vi "MGI Add Error[].vi"(8 "error in (no error)":errorcluster, 10 "Error[]":errorcluster[](array[cluster]), 11 "MGI Error Handler in":refnum<class "MGI Error Reporter Dialog.lvclass">) -> (0 "error out":errorcluster, 3 "MGI Error Handler out":refnum<class "MGI Error Reporter Dialog.lvclass">)   [LabVIEW 2016, in "MGI Error Reporter Dialog.lvclass"]
doc: "Add the errors in the specified array to the History Listbox. A child class may override this VI, which stores errors by process date and time (from most recent to oldest).\n\nAuthored by Shawn Walpole\nsupport@mooregoodideas.com\nwww.mooregoodideas.com\n\nCopyright (c) 2010, Moore Good Ideas, Inc.\n\nAll rights reserved.\n\nRedistribution and use in source and binary forms, with or without modification, are permitted provided that the following conditions are met:\n\n * Redistributions of source code must retain the above copyright notice, this list of conditions and the following disclaimer.\n * Redistributions in binary form must reproduce the above copyright notice, this list of conditions and the following disclaimer in the documentation and/or other materials provided with the distribution.\n * Neither the name of Moore Good Ideas, Inc. nor the names of its contributors may be used to endorse or promote products derived from this software without specific prior written permission.\n\nTHIS SOFTWARE IS PROVIDED BY THE COPYRIGHT HOLDERS AND CONTRIBUTORS \"AS IS\" AND ANY EXPRESS OR IMPLIED WARRANTIES, INCLUDING, BUT NOT LIMITED TO, THE IMPLIED WARRANTIES OF MERCHANTABILITY AND FITNESS FOR A PARTICULAR PURPOSE ARE DISCLAIMED. IN NO EVENT SHALL THE COPYRIGHT OWNER OR CONTRIBUTORS BE LIABLE FOR ANY DIRECT, INDIRECT, INCIDENTAL, SPECIAL, EXEMPLARY, OR CONSEQUENTIAL DAMAGES (INCLUDING, BUT NOT LIMITED TO, PROCUREMENT OF SUBSTITUTE GOODS OR SERVICES; LOSS OF USE, DATA, OR PROFITS; OR BUSINESS INTERRUPTION) HOWEVER CAUSED AND ON ANY THEORY OF LIABILITY, WHETHER IN CONTRACT, STRICT LIABILITY, OR TORT (INCLUDING NEGLIGENCE OR OTHERWISE) ARISING IN ANY WAY OUT OF THE USE OF THIS SOFTWARE, EVEN IF ADVISED OF THE POSSIBILITY OF SUCH DAMAGE."
uses:
  <userlib>/_MGI/Error Reporter/MGI Error Reporter Dialog/MGI Error Reporter Dialog.lvclass
  <userlib>/_MGI/Application Control/MGI Set Scrollbar/MGI Set Multicolumn Listbox Scrollbar.vi
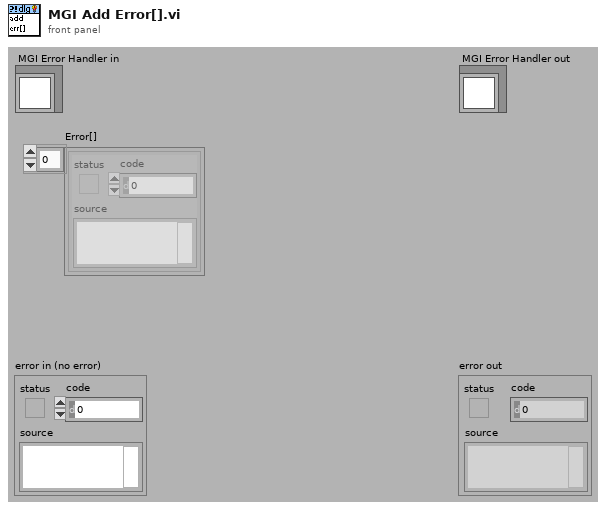
[diagram p1: front panel]
types:
  T1 = typedef "MGI Error Reporter Dialog.lvclass/MGI Dialog UI Refs Cluster.ctl" = cluster{"LB Ref":refnum<vi>, "Details Ref":refnum<vi>, "Caller Ring Ref":refnum<vi>, "Message Ref":refnum<vi>, "Clear Btn Ref":refnum<vi>}
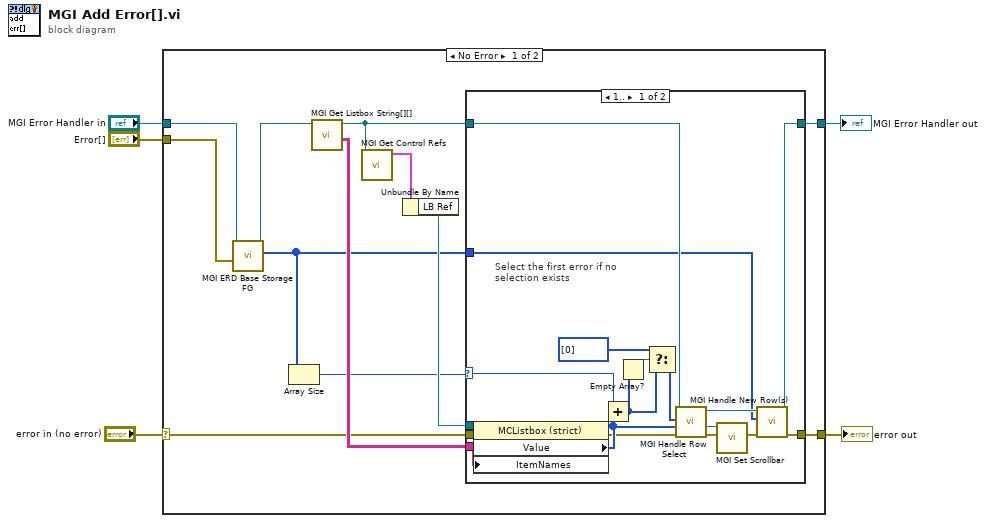
[diagram p0: block diagram]
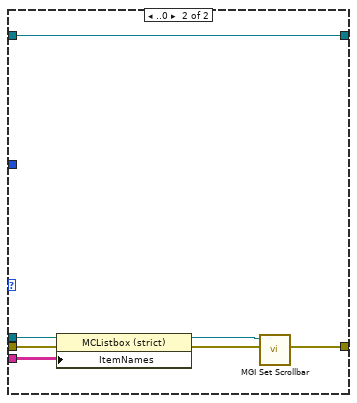
[diagram p2: hidden frame]
diagram:
  n1 = case shown="No Error" "error in (no error)" {
    selector: "error in (no error)" -> [w7 w43]
    tunnel: [w17 w43] -> w4
    tunnel: [w16 w42] -> w2
    tunnel: "MGI Error Handler in" -> [w14 w42]
    tunnel: "Error[]" -> [w15 _]
    frame No Error {
      n2 = call-dynamic "MGI ERD Base Storage FG.vi"("error[]"=w15, "MGI Error Reporter Dialog in"=w14) -> ("LB Row Inserted[]"=w6:i32[], "MGI Error Reporter Dialog Out"=w9:refnum<class "MGI Error Reporter Dialog.lvclass">)  [unwired: 2 in, 6 out]
      n3 = Array Size(array=w6) -> (size(s)=w10:i32)
      n4 = call-dynamic "MGI Get Listbox String[][].vi"("MGI Error Dialog in"=w9) -> ("Error[Row][Err/Warn,Name,Time,Count]"=w11:string[][], "MGI Error Dialog out"=w8:refnum<class "MGI Error Reporter Dialog.lvclass">)  [unwired: 2 in, 7 out]
      n5 = call <userlib>:"MGI Get Control Refs.vi"("MGI Error Dialog.lvclass"=w8) -> ("Refs"=w13:T1)  [unwired: 10 out]
      n6 = Unbundle By Name(w13) -> ("LB Ref"=w12:refnum<vi>)
      n7 = case shown="1.." w10 {
        selector: w10 -> [w27 _]
        tunnel: [w20 w36] -> w17
        tunnel: [w19 w35] -> w16
        tunnel: w7 -> [w34 w41]
        tunnel: w12 -> [w28 w38]
        tunnel: w11 -> [w30 w40]
        tunnel: w8 -> [w29 w35]
        tunnel: w6 -> [w18 _]
        frame 1.. {
          # "Select the first error if no selection exists"
          n8 = property class="MCListbox (strict)"(reference=w28, error in=w34, "ItemNames"=w30) -> (error out=w31:errorcluster, "Value"=w32:i32[])  [unwired: 1 out]
          n9 = Add(x=w27, y=w32) -> (x+y=w24:i32[])
          n10 = Empty Array?(array=w24) -> (empty?=w23:bool)
          n11 = Select(t=i32[] [0] ("Selected[]"), s=w23, f=w24) -> (s? t:f=w25:i32[])
          n12 = call-dynamic "MGI Handle Row Select.vi"("error in (no error)"=w31, "Old Selected[]"=w32, "Selected[]"=w25, "MGI Error Handler in"=w29) -> ("error out"=w33:errorcluster, "MGI Error Handler out"=w22:refnum<class "MGI Error Reporter Dialog.lvclass">)  [unwired: 6 out]
          n13 = call-poly <userlib>:"MGI Set Scrollbar.vi"("Error In"=w33, "Listbox Reference In"=w28) -> ("Error Out"=w21:errorcluster)  [unwired: 9 out]
          n14 = call-dynamic "MGI Handle New Row(s).vi"("error in (no error)"=w21, "NewRows[]"=w18, "Error Reporter Dialog in"=w22) -> ("error out"=w20:errorcluster, "Error Reporter Dialog out"=w19:refnum<class "MGI Error Reporter Dialog.lvclass">)  [unwired: 7 in]
        }
        frame ..0 {
          n15 = property class="MCListbox (strict)"(reference=w38, error in=w41, "ItemNames"=w40) -> (reference out=w37:refnum<vi>, error out=w39:errorcluster)
          n16 = call-poly <userlib>:"MGI Set Scrollbar.vi"("Error In"=w39, "Listbox Reference In"=w37) -> ("Error Out"=w36:errorcluster)  [unwired: 9 out]
        }
      }
    }
    frame Error {
    }
  }
  "error out" <- w4
  "MGI Error Handler out" <- w2
